vi "Data Power Output.vi"(8 "error in (no error)":errorcluster, 11 "RS Z2X in":refnum<class "RS Z2X.lvclass">) -> (0 "error out":errorcluster, 2 "Power Out":dbl, 3 "RS Z2X out":refnum<class "RS Z2X.lvclass">)   [LabVIEW 2020, in "RS Z2X.lvclass"]
uses:
  RS Z2X.lvclass
  C:/Sandbox/RF Bench/Source Code/WiSpry Test Framework/Instruments/Instrument.lvclass
  Instrument.lvclass/Instrument.ctl
  Instrument.lvclass
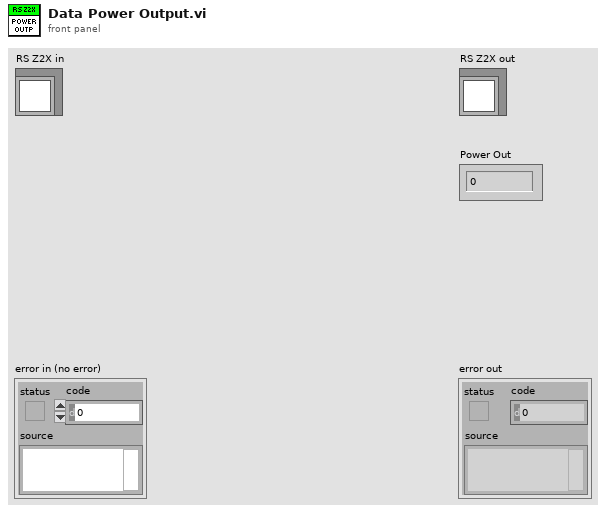
[diagram p1: front panel]
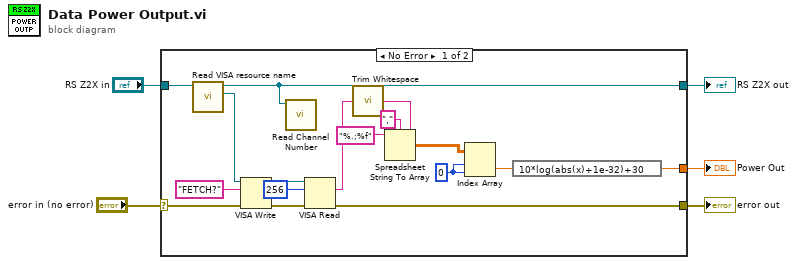
[diagram p0: block diagram]
diagram:
  n1 = case shown="No Error" "error in (no error)" {
    selector: "error in (no error)" -> [w20 w24]
    tunnel: "RS Z2X in" -> [w22 w23]
    tunnel: [w7 _] -> w3
    tunnel: [w9 w24] -> w2
    tunnel: [w6 w23] -> w1
    frame No Error {
      w10 = 0 ("disabled index (col)")
      n2 = call "Read VISA resource name.vi"("Instrument in"=w22) -> ("VISA resource name"=w21:refnum<visa-resource-name>, "Instrument out"=w6:refnum<class "RS Z2X.lvclass">)  [unwired: 9 in]
      n3 = VISA Write(VISA resource name=w21, write buffer="FETCH?", error in (no error)=w20) -> (VISA resource name out=w17:refnum<visa-resource-name>, error out=w18:errorcluster)  [unwired: 1 out]
      n4 = call-dynamic "Read Channel Number.vi"("Power Meter in"=w6) -> ()  [unwired: 9 in, 2 out]
      n5 = VISA Read(VISA resource name=w17, byte count=u32 256, error in (no error)=w18) -> (read buffer=w15:string, error out=w9:errorcluster)  [unwired: 2 out]
      n6 = call <vilib>:"Trim Whitespace.vi"("string"=w15) -> ("trimmed string"=w12:string)  [unwired: 1 in]
      n7 = Spreadsheet String To Array(delimiter (Tab)=",", format string="%.;%f", spreadsheet string=w12) -> (array=w11:dbl[][])  [unwired: 1 in]
      n8 = Index Array(array=w11, index (row)=w10, index (col)=w10) -> (element=w8:dbl)
      n9 = expression code="10*log(abs(x)+1e-32)+30"(w8) -> (w7:dbl)
    }
    frame Error {
    }
  }
  "error out" <- w2
  "RS Z2X out" <- w1
  "Power Out" <- w3
